vi "solar_misc CPU.vi"(8 "error in (no error)":errorcluster, 9 "Close Refnums? (F)":bool) -> (0 "error out":errorcluster, 3 "CPU_USAGE":T1 {"UPTIME_SEC" format="%#f"; "CPU8" format="%#f"; "CPU7" format="%#f"; "CPU6" format="%#f"; "CPU5" format="%#f"; "CPU4" format="%#f"; "CPU3" format="%#f"; "CPU2" format="%#f"; "CPU1" format="%#f"; "CPU_TOTAL" format="%#f"; "MEMORY_USED" format="%#f"; "AVAILABLE_MB" format="%#f"; "FREE_MB" format="%#f"; "COMMITTED_MB" format="%#f"})   [LabVIEW 2018]
doc: "This returns the CPU memory and processor utilitization using the .NET System.Diagnostics.PerformanceCounter API."
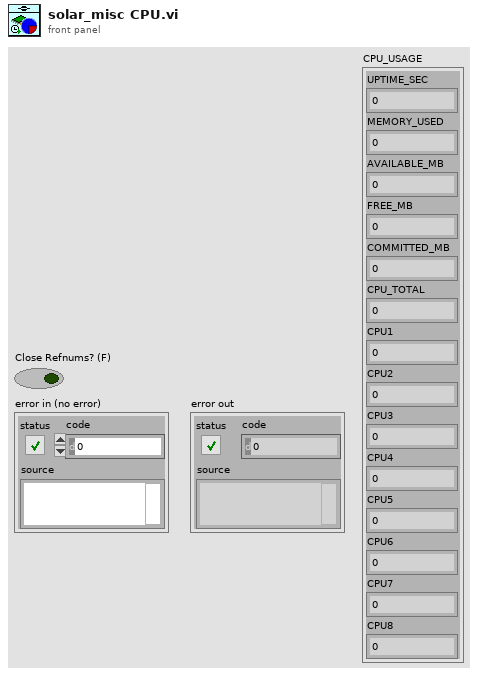
[diagram p1: front panel]
types:
  T1 = cluster{"UPTIME_SEC":dbl, "MEMORY_USED":dbl, "AVAILABLE_MB":dbl, "FREE_MB":dbl, "COMMITTED_MB":dbl, "CPU_TOTAL":dbl, "CPU1":dbl, "CPU2":dbl, "CPU3":dbl, "CPU4":dbl, "CPU5":dbl, "CPU6":dbl, "CPU7":dbl, "CPU8":dbl}
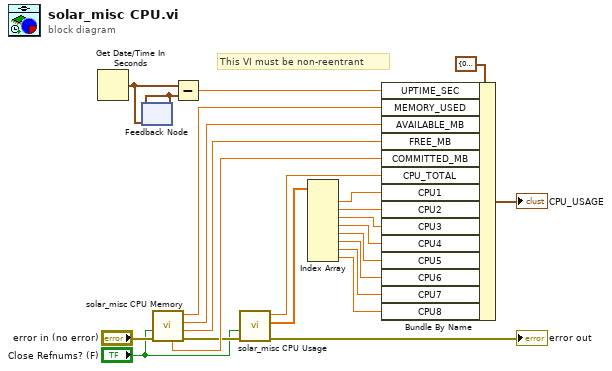
[diagram p0: block diagram]
diagram:
  # "This VI must be non-reentrant"
  n1 = Get Date/Time In Seconds() -> (seconds since 1Jan1904=w15:timestamp)
  n2 = feedback #1(w15) -> (w14:timestamp)
  n3 = feedback-in #1(w14) -> ()
  n4 = call "solar_misc CPU Memory.vi"("error in (no error)"="error in (no error)", "Close Refnums? (F)"="Close Refnums? (F)") -> ("error out"=w17:errorcluster, "Free (MB)"=w21:dbl, "Available (MB)"=w20:dbl, "Memory Usage (%)"=w19:dbl, "Committed (MB)"=w22:dbl)  [unwired: 5 in]
  n5 = Subtract(x=w15, y=w14) -> (x-y=w13:dbl)
  n6 = call "solar_misc CPU Usage.vi"("error in (no error)"=w17, "Close Refnums? (F)"="Close Refnums? (F)") -> ("error out"=→"error out":errorcluster, "Processor CPU Usage (%)"=w11:dbl[], "Total CPU Usage (%)"=w12:dbl)  [unwired: 7 in]
  n7 = Index Array(array=w11) -> (element #1=w10:dbl, element #2=w9:dbl, element #3=w8:dbl, element #4=w7:dbl, element #5=w6:dbl, element #6=w5:dbl, element #7=w4:dbl, element #8=w3:dbl)  [unwired: 8 in]
  n8 = Bundle By Name(cluster=T1 {"UPTIME_SEC"=0.0, "MEMORY_USED"=0.0, "AVAILABLE_MB"=0.0, "FREE_MB"=0.0, "COMMITTED_MB"=0.0, "CPU_TOTAL"=0.0, "CPU1"=0.0, "CPU2"=0.0, "CPU3"=0.0, "CPU4"=0.0, "CPU5"=0.0, "CPU6"=0.0, "CPU7"=0.0, "CPU8"=0.0} ("ICATS_CPU_USAGE"), "UPTIME_SEC"=w13, "MEMORY_USED"=w19, "AVAILABLE_MB"=w20, "FREE_MB"=w21, "COMMITTED_MB"=w22, "CPU_TOTAL"=w12, "CPU1"=w10, "CPU2"=w9, "CPU3"=w8, "CPU4"=w7, "CPU5"=w6, "CPU6"=w5, "CPU7"=w4, "CPU8"=w3) -> (→"CPU_USAGE":T1)
